vi "PollHexStatus.vi"(8 "error in (no error)":errorcluster, 11 "System no.":i32) -> (0 "error out":errorcluster, 3 "Status Cluster 2":T1)   [LabVIEW 2020, in "C-887.lvclass"]
uses:
  C-887.lvclass
panel:
  in  "Status Cluster":T1
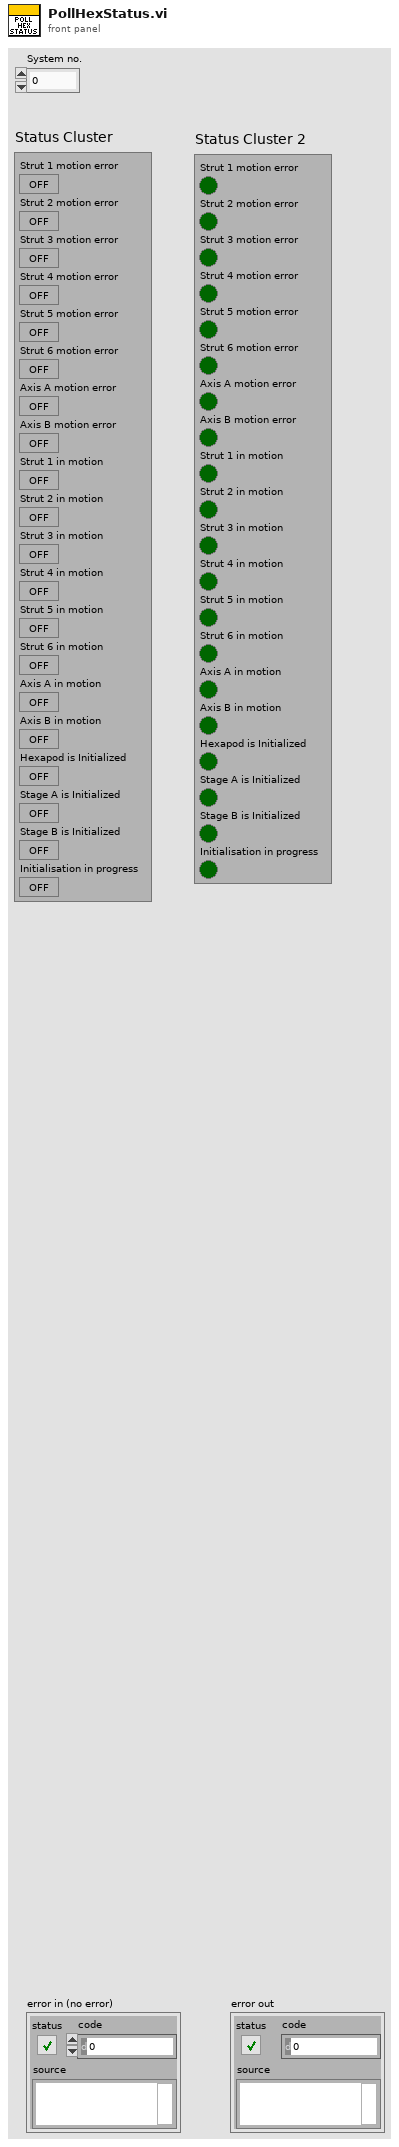
[diagram p1: front panel]
types:
  T1 = cluster{"Strut 1 motion error":bool, "Strut 2 motion error":bool, "Strut 3 motion error":bool, "Strut 4 motion error":bool, "Strut 5 motion error":bool, "Strut 6 motion error":bool, "Axis A motion error":bool, "Axis B motion error":bool, "Strut 1 in motion":bool, "Strut 2 in motion":bool, "Strut 3 in motion":bool, "Strut 4 in motion":bool, "Strut 5 in motion":bool, "Strut 6 in motion":bool, "Axis A in motion":bool, "Axis B in motion":bool, "Hexapod is Initialized":bool, "Stage A is Initialized":bool, "Stage B is Initialized":bool, "Initialisation in progress":bool}
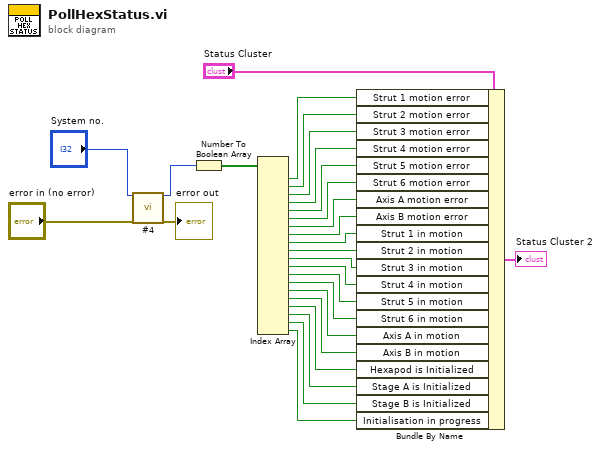
[diagram p0: block diagram]
diagram:
  n1 = call "#4.vi"("System no."="System no.", "error in"="error in (no error)") -> ("Status information"=w27:i32, "error out"=→"error out":errorcluster)  [unwired: 15 in, 1 out]
  n2 = Number To Boolean Array(number=w27) -> (Boolean array=w26:bool[])
  n3 = Index Array(array=w26) -> (element #1=w4:bool, element #2=w5:bool, element #3=w6:bool, element #4=w7:bool, element #5=w8:bool, element #6=w9:bool, element #7=w10:bool, element #8=w11:bool, element #9=w12:bool, element #10=w13:bool, element #11=w14:bool, element #12=w15:bool, element #13=w16:bool, element #14=w17:bool, element #15=w18:bool, element #16=w19:bool, element #17=w20:bool, element #18=w21:bool, element #19=w22:bool, element #20=w23:bool)  [unwired: 20 in]
  n4 = Bundle By Name(cluster="Status Cluster", "Strut 1 motion error"=w4, "Strut 2 motion error"=w5, "Strut 3 motion error"=w6, "Strut 4 motion error"=w7, "Strut 5 motion error"=w8, "Strut 6 motion error"=w9, "Axis A motion error"=w10, "Axis B motion error"=w11, "Strut 1 in motion"=w12, "Strut 2 in motion"=w13, "Strut 3 in motion"=w14, "Strut 4 in motion"=w15, "Strut 5 in motion"=w16, "Strut 6 in motion"=w17, "Axis A in motion"=w18, "Axis B in motion"=w19, "Hexapod is Initialized"=w20, "Stage A is Initialized"=w21, "Stage B is Initialized"=w22, "Initialisation in progress"=w23) -> (→"Status Cluster 2":T1)
